vi "Get VI Checksums.vi"(8 "error in (no error)":errorcluster, 11 "SDIST in":refnum<class "NI_AB_API_SDIST.lvclass">) -> (0 "error out":errorcluster, 2 "VI Checksums":string[](array[string]), 3 "SDIST out":refnum<class "NI_AB_API_SDIST.lvclass">, 5 "Has errors?":bool)   [LabVIEW 2020, in "NI_AB_API_SDIST.lvclass"]
uses:
  <vilib>/AppBuilder/AB_API/SDIST/NI_AB_API_SDIST.lvclass
  <vilib>/AppBuilder/AB_API/Build/NI_AB_API_Build.lvclass
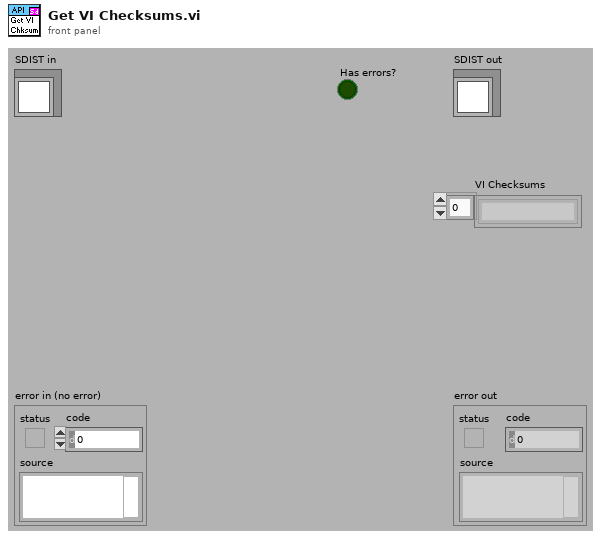
[diagram p1: front panel]
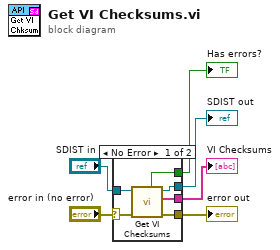
[diagram p0: block diagram]
diagram:
  n1 = case shown="No Error" "error in (no error)" {
    selector: "error in (no error)" -> [w9 w14]
    tunnel: [w10 w14] -> w5
    tunnel: [w11 w13] -> w3
    tunnel: "SDIST in" -> [w12 w13]
    tunnel: [w8 _] -> w2
    tunnel: [w7 _] -> w1
    frame No Error {
      n2 = call-parent "Get VI Checksums.vi"("error in (no error)"=w9, "NI_AB_API_Build in"=w12) -> ("error out"=w10:errorcluster, "VI Checksums"=w8:string[], "NI_AB_API_Build out"=w11:refnum<class "NI_AB_API_SDIST.lvclass">, "Has errors?"=w7:bool)  [unwired: 6 in]
    }
    frame Error {
    }
  }
  "error out" <- w5
  "SDIST out" <- w3
  "Has errors?" <- w1
  "VI Checksums" <- w2
